vi "WLC Fitting_Final_v2_YCC.vi"(3 "initial parameters (Lp,Lc) or (Lc,K)":dbl[](array[numeric])=[40.0, 1150.0], 4 "Fitting Cluster":T1={"cr (um)"=0.0, "yr (V)"=0.0, "trap height(nm)"=300.0, "bead radius(nm)"=515.0, "Length offset"=550.0, "Upper Force(pN)"=500.0, "cr shift (nm)"=0.0, "yr shift (mV)"=0.0, "LaserPower (mW)"=1200.0, "conversion factor (V/um)"=0.0, "Stiffness (pN/nm)"=0.0, "xDNA cut outside"=3000.0, "Lower Force(pN)"=5.0, "c for zbd"=0.0}, 5 "Enum":T2(ring), 6 "Load Stage-QPD data":path, 7 "T=Fit U or twoside\nF=Fit F":bool=TRUE, 8 "F+U data?":bool, 9 "Finish Fitting":bool, 10 "Ready to Fit":bool, 11 "DataRecord type":enum32{"OneDirectionOnly?", "TwoSide Data"}(tab)) -> (0 "best fit parameters":dbl[](array[numeric]), 1 "r^2":dbl)   [LabVIEW 2014]
uses:
  <vilib>/gmath/NI_Gmath.lvlib
  <vilib>/gmath/NumericalOptimization/Nonlinear Curve Fit LM formula string.vi
  <vilib>/Utility/file.llb/Write To Spreadsheet File (DBL).vi
  <vilib>/Utility/file.llb/Read From Spreadsheet File (DBL).vi
  SubVI/WLC-Fitting Cluster.ctl
panel:
  in  "Given Lp (nm)":dbl=5.0
  in  "Lower Force (pN)":dbl=6.0
  in  "Upper Force (pN)":dbl=45.0
  in  "Set lower foce offset?":bool
  out "U-Force or twoside 2":dbl[](array[numeric])
  out "U-xDNA or twoside 2":dbl[](array[numeric])
  in  "initial guess K (pN)":dbl=1200.0
  out "OneDirectionOnly?":bool=TRUE
  in  "Fit \"+\"(RHS) ?":bool=TRUE
  in  "Fit One Side?":bool
  in  "Reverse sign?":bool=TRUE
  out "Cut-Force for eWLC (pN)":dbl[](array[numeric])
  out "best nonlinear fit extension (eWLC)":dbl[](array[numeric])
  in  "T=use stuckbead 7th order\nF=use slope 1st order calibrate":bool
  out "Force to be saved":dbl[](array[numeric])
  out "xDNA to be saved":dbl[](array[numeric])
  out "F-Force":dbl[](array[numeric])
  out "F-xDNA":dbl[](array[numeric])
  in  "F-yr shift (mV)":dbl
  in  "F-cr shift (nm)":dbl
  out "F-QPD signal (V)":dbl[](array[numeric])
  out "F-Stage Positions (um)":dbl[](array[numeric])
  in  "stuckbead path (dialog if empty)":path=path "D:/Calibration-Stuckbead-Scan/20181220/2/202224-x-Stuckbead Scan-6000.00-step 5.00 nm-QPD height 3.340-h0.txt"
  out "Save to Path":path
  out "best nonlinear fit force (M-S)":dbl[](array[numeric])
  in  "SaveName":enum16{"ForecExtension Only", "WLC Fitting"}(ring)
  in  "Save Calibrated Data?":bool
  out "U-Force or twoside":dbl[](array[numeric])
  out "U-xDNA or twoside":dbl[](array[numeric])
  out "Fitting Cluster for indicator":T1={"cr (um)"=0.0, "yr (V)"=0.0, "trap height(nm)"=0.0, "bead radius(nm)"=520.0, "Length offset"=0.0, "Upper Force(pN)"=0.0, "cr shift (nm)"=0.0, "yr shift (mV)"=0.0, "LaserPower (mW)"=0.0, "conversion factor (V/um)"=0.0, "Stiffness (pN/nm)"=0.0154, "xDNA cut outside"=0.0, "Lower Force(pN)"=5.0, "c for zbd"=0.0}
  in  "Tab Control":T3(tab)
  out "Stage-QPD Graph":T4(graph)
  out "U-Extension-Force Graph":cluster{"xDNA":dbl[], "Force":dbl[]}(graph)
  out "F-Extension-Force Graph":cluster{"xDNA":dbl[], "Force":dbl[]}(graph)
  out "All-Extension-Force Graph":T5(graph)
  out "Extension-Force and WLC Graph":cluster{"xDNA":dbl[], "Force":dbl[]}[](graph)
  out "All Extension-Force and WLC Graph":T6(graph)
  out "Cut Stage Position (um)":dbl[](array[numeric])
  out "Cut QPD (V)":dbl[](array[numeric])
  in  "Delete Outside Signal?":bool
  out "U-QPD signal or All QPD  (V)":dbl[](array[numeric])
  out "U-Stage Positions or All stage positions (um)":dbl[](array[numeric])
  in  "QPD":dbl[](array[numeric])
  in  "Stage":dbl[](array[numeric])
  in  "T=Read data mode?\nF=Real time fit":bool=TRUE
  # "5180bp=1750.8 nm\n3281bp=1109.0 nm"
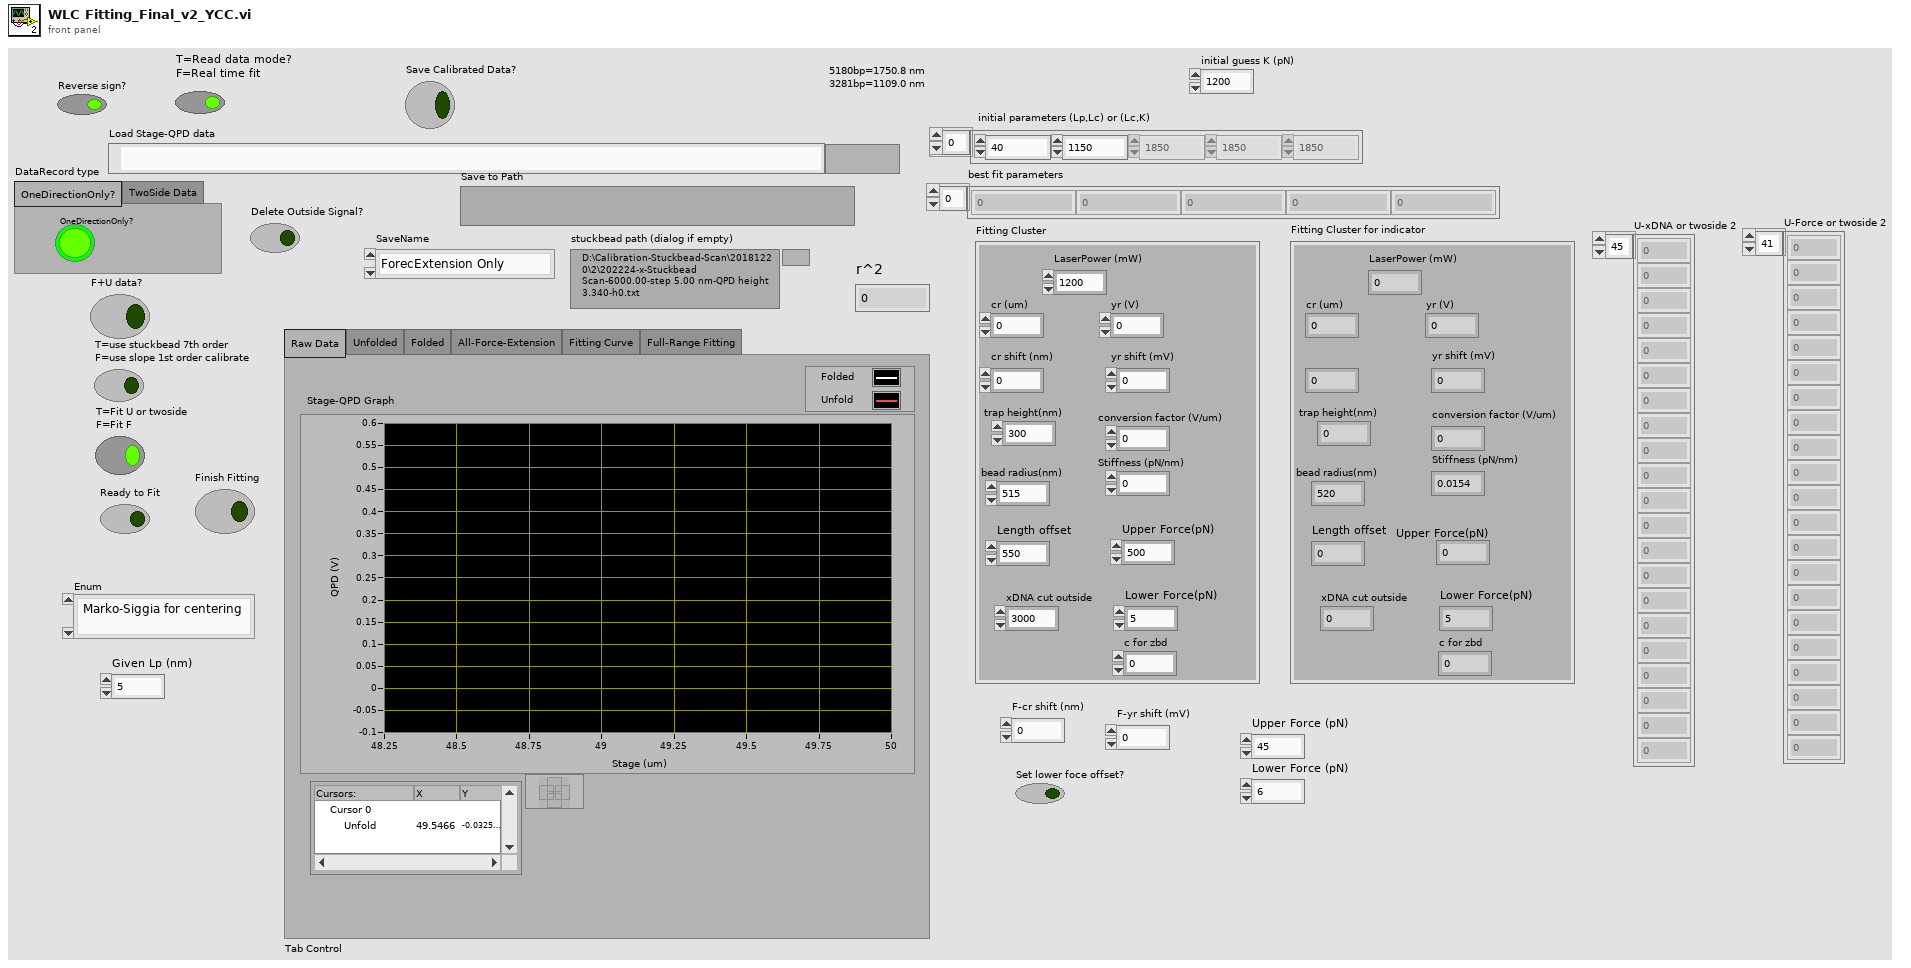
[diagram p1: front panel]
types:
  T1 = typedef "WLC-Fitting Cluster.ctl" = cluster{"cr (um)":dbl, "yr (V)":dbl, "trap height(nm)":dbl, "bead radius(nm)":dbl, "Length offset":dbl, "Upper Force(pN)":dbl, "cr shift (nm)":dbl, "yr shift (mV)":dbl, "LaserPower (mW)":dbl, "conversion factor (V/um)":dbl, "Stiffness (pN/nm)":dbl, "xDNA cut outside":dbl, "Lower Force(pN)":dbl, "c for zbd":dbl}
  T2 = enum16{" Marko-Siggia for centering", "Marko-Siggia", "direct fit (Lp,Lc,K)", "fit K (Lp,Lc,K)", "eWLC (Lp=45,Lc,K)"}
  T3 = enum32{"Raw Data", "Unfolded", "Folded", "All-Force-Extension", "Fitting Curve", "Full-Range Fitting"}
  T4 = cluster{"Sorted Stage Position (um)":dbl[], "Sorted QPD (V)":dbl[]}[]
  T5 = cluster{"Folded-xDNA":dbl[], "Folded-Force":dbl[]}[]
  T6 = cluster{"cut-full xDNA":dbl[], "cut-full Force":dbl[]}[]
  T7 = cluster{"model":string, "Parameters":string[], "x":string}
  T8 = cluster{"F-Stage Positions (um) ":dbl[], "F-QPD signal (V) ":dbl[]}
  T9 = cluster{"U-Stage Positions or All stage positions (um)":dbl[], "U-QPD signal or All QPD  (V)":dbl[]}
  T10 = cluster{"U-Stage Positions or All stage positions (um)":dbl[], "U-QPD signal or All QPD  (V)":dbl[]}[]
  T11 = cluster{"Folded-xDNA":dbl[], "Folded-xDNA":dbl[]}
  T12 = cluster{"cut-full xDNA":dbl[], "best nonlinear fit":dbl[]}
  T13 = cluster{"best nonlinear fit":dbl[], "cut-full Force":dbl[]}
  T14 = cluster{"cut-full xDNA":dbl[], "cut-full Force":dbl[]}
  T15 = cluster{"Fit Extension (nm)":dbl[], "Fit Force (pN)":dbl[]}
  T16 = cluster{"xDNA to be saved":dbl[], "Force to be saved":dbl[]}
  T17 = cluster{"xDNA to be saved":dbl[], "Force to be saved":dbl[]}[]
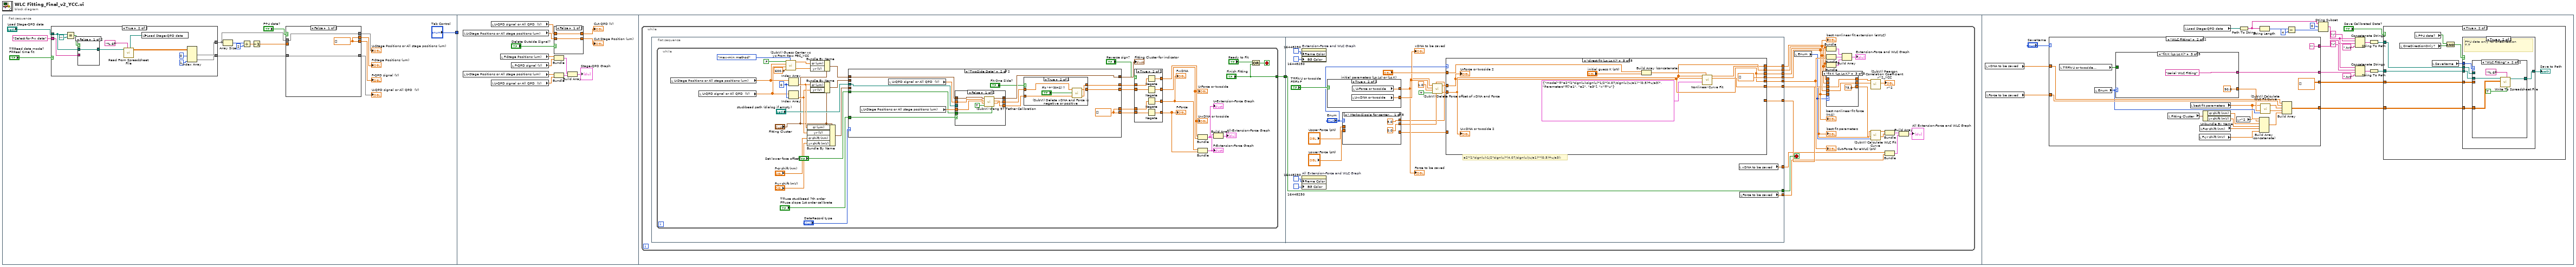
[diagram p0: block diagram]
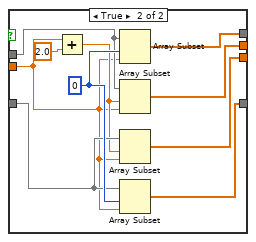
[diagram p2: hidden frame]
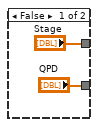
[diagram p3: hidden frame]
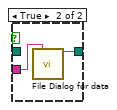
[diagram p4: hidden frame]
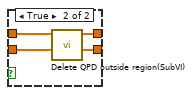
[diagram p5: hidden frame]
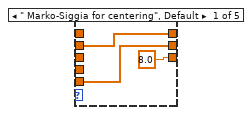
[diagram p6: hidden frame]
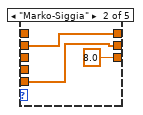
[diagram p7: hidden frame]
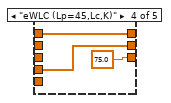
[diagram p8: hidden frame]
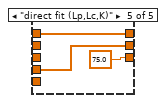
[diagram p9: hidden frame]
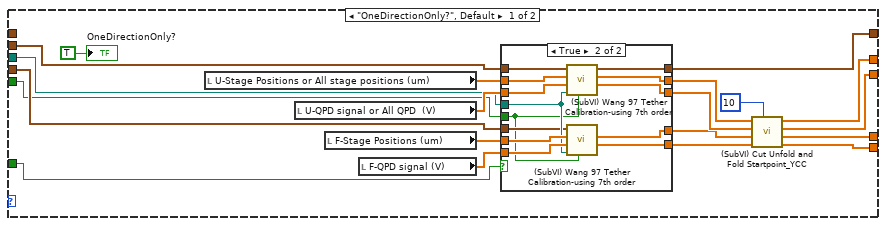
[diagram p11: hidden frame]
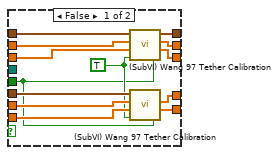
[diagram p12: hidden frame]
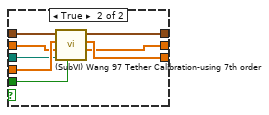
[diagram p14: hidden frame]
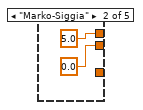
[diagram p15: hidden frame]
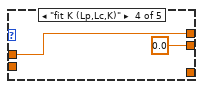
[diagram p17: hidden frame]
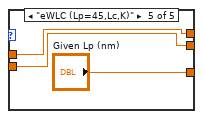
[diagram p18: hidden frame]
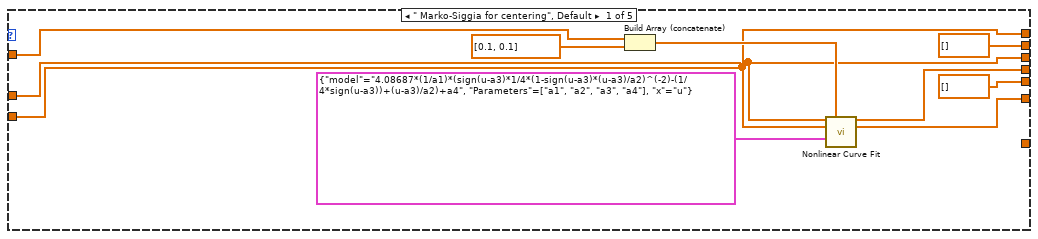
[diagram p19: hidden frame]
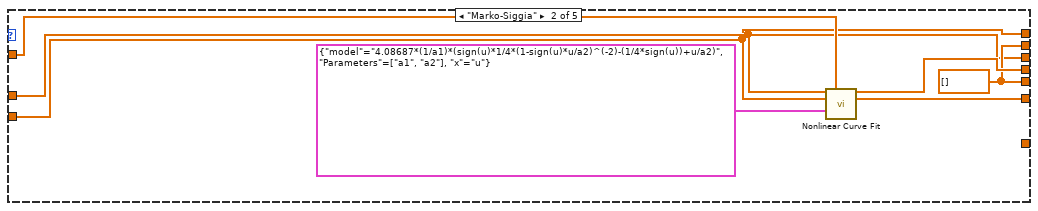
[diagram p20: hidden frame]
diagram:
  n1 = flat-sequence {
    tunnel: ["Tab Control"] -> w1
    tunnel: w1 -> [_]
    frame #0 {
      n2 = case shown="True" "T=Read data mode?\nF=Real time fit" {
        tunnel: ["QPD" w39] -> w11
        tunnel: ["Stage" w40] -> w6
        tunnel: "Select for F-x data" ("default name") -> [_ w36]
        tunnel: "Load Stage-QPD data" -> [_ w33]
        frame False {
        }
        frame True {
          n3 = Equal?(x=w33, y=path "") -> (x = y?=w34:bool)
          n4 = case shown="False" w34 {
            tunnel: [w44 w45] -> w37
            tunnel: w36 -> [_ w46]
            tunnel: w33 -> [w44 _]
            frame False {
            }
            frame True {
              n5 = call "File Dialog for data"("prompt"=w46) -> ("selected path"=w45:path)  [unwired: 11 in, 3 out]
            }
          }
          n6 = call-poly <vilib>:"Read From Spreadsheet File.vi"("format (%.3f)"="%.6f", "file path (dialog if empty)"=w37) -> ("all rows"=w43:dbl[][], "new file path (Not A Path if cancelled)"=w32:path)  [unwired: 5 in, 3 out]
          n7 = local write "Load Stage-QPD data"(w32) -> ()
          n8 = Index Array(array=w43, index (col) #1=0 ("disabled index (col)"), index (col) #2=1 ("index (col)")) -> (element #1=w40:dbl[], element #2=w39:dbl[])  [unwired: 2 in]
        }
      }
      n9 = Array Size(array=w6) -> (size(s)=w7:i32)
      n10 = Divide(x=w7, y=2) -> (x/y=w5:dbl)
      n11 = Decrement(x=w5) -> (x-1=w4:dbl)
      n12 = case shown="False" "F+U data?" {
        tunnel: w6 -> [w19 w25]
        tunnel: w11 -> [w18 w26]
        tunnel: [w19 w29] -> w10
        tunnel: [w18 w27] -> w9
        tunnel: w4 -> [_ w20]
        tunnel: [w17 w24] -> w3
        tunnel: [w17 w23] -> w2
        frame False {
          w17 = dbl[] []
        }
        frame True {
          w28 = 0 ("index")
          n13 = Add(x=w20, y=2.0) -> (x+y=w21:dbl)
          n14 = Array Subset(array=w25, index=w28, length=w20) -> (w29:dbl[])
          n15 = Array Subset(array=w25, index=w21, length=w20) -> (w24:dbl[])
          n16 = Array Subset(array=w26, index=w21, length=w20) -> (w23:dbl[])
          n17 = Array Subset(array=w26, index=w28, length=w20) -> (w27:dbl[])
        }
      }
      "U-Stage Positions or All stage positions (um)" <- w10
      "U-QPD signal or All QPD  (V)" <- w9
      "F-Stage Positions (um)" <- w3
      "F-QPD signal (V)" <- w2
    }
    frame #1 {
      n18 = local read "U-Stage Positions or All stage positions (um)"() -> (w57:dbl[])
      n19 = local read "U-Stage Positions or All stage positions (um)"() -> (w55:dbl[])
      n20 = local read "U-QPD signal or All QPD  (V)"() -> (w56:dbl[])
      n21 = local read "U-QPD signal or All QPD  (V)"() -> (w54:dbl[])
      n22 = local read "F-Stage Positions (um)"() -> (w48:dbl[])
      n23 = local read "F-QPD signal (V)"() -> (w47:dbl[])
      n24 = case shown="False" "Delete Outside Signal?" {
        tunnel: w56 -> [w60 w64]
        tunnel: w57 -> [w59 w63]
        tunnel: [w60 w62] -> w49
        tunnel: [w59 w61] -> w50
        frame False {
        }
        frame True {
          n25 = call "Delete QPD outside region(SubVI).vi"("Position Array In"=w63, "QPD signal In"=w64) -> ("Position Array Out"=w61:dbl[], "QPD signal Out"=w62:dbl[])  [unwired: 8 in]
        }
      }
      "Cut QPD (V)" <- w49
      "Cut Stage Position (um)" <- w50
      n26 = Bundle("F-Stage Positions (um)"=w48, "F-QPD signal (V)"=w47) -> (w53:T8)  [unwired: 1 in]
      n27 = Bundle("U-Stage Positions or All stage positions (um)"=w55, "U-QPD signal or All QPD  (V)"=w54) -> (w52:T9)  [unwired: 1 in]
      n28 = Build Array(w53, w52) -> (→"Stage-QPD Graph":T10)
    }
    frame #2 {
      n29 = while {
        stop <- w79 stop-if-true
        n30 = flat-sequence {
          tunnel: [w105] -> w80
          tunnel: [w262] -> w85
          tunnel: [w261] -> w76
          tunnel: [w259] -> w82
          tunnel: [w258] -> w86
          tunnel: [w257] -> w81
          tunnel: [w256] -> w88
          tunnel: [w255] -> w79
          tunnel: w80 -> [w255]
          tunnel: [w242] -> w77
          tunnel: [w241] -> w68
          tunnel: [w240] -> w67
          frame #0 {
            n31 = while {
              tunnel: ["Finish Fitting"] -> w105
              stop <- w109 stop-if-true
              w141 = 0 ("index")
              n32 = local read "U-Stage Positions or All stage positions (um)"() -> (w130:dbl[])
              n33 = local read "U-QPD signal or All QPD  (V)"() -> (w129:dbl[])
              n34 = call "(SubVI) Guess Center xc yc From Raw FEC_YCC.vi"("Read data?"=FALSE, "Enum"=enum16{"parity method", "max-min method"}."max-min method", "Stage array(um)"=w130, "QPD array (V)"=w129, "avg range for QPD center (nm)"=600.0) -> ("Guess-stage-center (um)"=w128:dbl, "Guess-QPD-center (V)"=w127:dbl)  [unwired: 2 in]
              n35 = Index Array(array=w130, index=w141) -> (element=w138:dbl)
              n36 = Index Array(array=w129, index=w141) -> (element=w137:dbl)
              n37 = Bundle By Name(cluster="Fitting Cluster", "cr (um)"=w138, "yr (V)"=w137, "cr shift (nm)"="F-cr shift (nm)", "yr shift (mV)"="F-yr shift (mV)") -> (w134:T1)
              n38 = Bundle By Name(cluster="Fitting Cluster", "cr (um)"=w128, "yr (V)"=w127) -> (w126:T1)
              n39 = Bundle By Name(cluster="Fitting Cluster", "cr (um)"=w138, "yr (V)"=w137) -> (w140:T1)
              n40 = case shown="\"TwoSide Data\"" "DataRecord type" {
                tunnel: w140 -> [w171 _]
                tunnel: [w172 w209] -> w139
                tunnel: w134 -> [w167 _]
                tunnel: w126 -> [_ w212]
                tunnel: [w161 w202] -> w123
                tunnel: [w160 w201] -> w117
                tunnel: [w159 w208] -> w122
                tunnel: [w158 w208] -> w121
                tunnel: "T=use stuckbead 7th order\nF=use slope 1st order calibrate" -> [w157 w207]
                tunnel: "stuckbead path (dialog if empty)" -> [w156 w206]
                tunnel: "Set lower foce offset?" -> [w154 w200]
                frame "OneDirectionOnly?", Default {
                  n41 = local read "U-Stage Positions or All stage positions (um)"() -> (w170:dbl[])
                  n42 = local read "U-QPD signal or All QPD  (V)"() -> (w173:dbl[])
                  n43 = local read "F-Stage Positions (um)"() -> (w169:dbl[])
                  n44 = local read "F-QPD signal (V)"() -> (w168:dbl[])
                  n45 = case shown="True" w157 {
                    tunnel: w173 -> [w185 w199]
                    tunnel: [w184 w198] -> w172
                    tunnel: w171 -> [w176 w197]
                    tunnel: w170 -> [w186 w196]
                    tunnel: w169 -> [w182 w195]
                    tunnel: w168 -> [w181 w194]
                    tunnel: w156 -> [_ w193]
                    tunnel: w167 -> [w183 w192]
                    tunnel: [w180 w191] -> w165
                    tunnel: [w179 w190] -> w164
                    tunnel: [w178 w189] -> w163
                    tunnel: [w177 w188] -> w162
                    tunnel: w154 -> [w174 w187]
                    frame False {
                      w175 = TRUE ("X=T\nY=F")
                      n46 = call "(SubVI) Wang 97 Tether Calibration.vi"("Set lower foce offset?"=w174, "X=T\nY=F"=w175, "QPD signal"=w185, "Stage Position"=w186, "Fitting Cluster"=w176) -> ("Force"=w179:dbl[], "xDNA"=w180:dbl[], "output cluster"=w184:T1)
                      n47 = call "(SubVI) Wang 97 Tether Calibration.vi"("Set lower foce offset?"=w174, "X=T\nY=F"=w175, "QPD signal"=w181, "Stage Position"=w182, "Fitting Cluster"=w183) -> ("Force"=w177:dbl[], "xDNA"=w178:dbl[])  [unwired: 1 out]
                    }
                    frame True {
                      n48 = call "(SubVI) Wang 97 Tether Calibration-using 7th order.vi"("Set lower foce offset?"=w187, "stuckbead path (dialog if empty)"=w193, "QPD signal"=w199, "Stage Position"=w196, "Fitting Cluster"=w197) -> ("Force"=w190:dbl[], "xDNA"=w191:dbl[], "output cluster"=w198:T1)  [unwired: 2 in, 2 out]
                      n49 = call "(SubVI) Wang 97 Tether Calibration-using 7th order.vi"("Set lower foce offset?"=w187, "stuckbead path (dialog if empty)"=w193, "QPD signal"=w194, "Stage Position"=w195, "Fitting Cluster"=w192) -> ("Force"=w188:dbl[], "xDNA"=w189:dbl[])  [unwired: 2 in, 3 out]
                    }
                  }
                  n50 = call "(SubVI) Cut Unfold and Fold Startpoint_YCC.vi"("number to cut"=10, "Folded-Force in"=w162, "Folded-xDNA in"=w163, "Unfolded-Force"=w164, "Unfolded-xDNA"=w165) -> ("Folded-Force"=w158:dbl[], "Folded-xDNA"=w159:dbl[], "Unfolded-Force"=w160:dbl[], "Unfolded-xDNA"=w161:dbl[])  [unwired: 3 in]
                  "OneDirectionOnly?" <- TRUE
                }
                frame "TwoSide Data" {
                  w208 = dbl[] [] ("Folded-xDNA")
                  n51 = local read "U-Stage Positions or All stage positions (um)"() -> (w211:dbl[])
                  n52 = local read "U-QPD signal or All QPD  (V)"() -> (w210:dbl[])
                  n53 = case shown="False" w207 {
                    tunnel: w212 -> [w227 w235]
                    tunnel: w211 -> [w226 w234]
                    tunnel: w210 -> [w225 w233]
                    tunnel: [w224 w231] -> w209
                    tunnel: [w223 w230] -> w203
                    tunnel: [w222 w229] -> w204
                    tunnel: w206 -> [_ w232]
                    tunnel: w200 -> [w220 w228]
                    frame False {
                      n54 = call "(SubVI) Wang 97 Tether Calibration.vi"("Set lower foce offset?"=w220, "X=T\nY=F"=TRUE ("X=T\nY=F"), "QPD signal"=w225, "Stage Position"=w226, "Fitting Cluster"=w227) -> ("Force"=w222:dbl[], "xDNA"=w223:dbl[], "output cluster"=w224:T1)
                    }
                    frame True {
                      n55 = call "(SubVI) Wang 97 Tether Calibration-using 7th order.vi"("Set lower foce offset?"=w228, "stuckbead path (dialog if empty)"=w232, "QPD signal"=w233, "Stage Position"=w234, "Fitting Cluster"=w235) -> ("Force"=w229:dbl[], "xDNA"=w230:dbl[], "output cluster"=w231:T1)  [unwired: 2 in, 2 out]
                    }
                  }
                  n56 = case shown="True" "Fit One Side?" {
                    tunnel: w204 -> [w214 w218]
                    tunnel: w203 -> [w213 w217]
                    tunnel: [w213 w216] -> w202
                    tunnel: [w214 w215] -> w201
                    frame False {
                    }
                    frame True {
                      n57 = call "(SubVI) Delete xDNA and Force is negative or positive.vi"("xDNA"=w217, "T=positive (RHS)\nF=negative (LHS)"="Fit \"+\"(RHS) ?", "Force"=w218) -> ("xDNA-cut"=w216:dbl[], "Force-cut"=w215:dbl[])  [unwired: 1 in]
                    }
                  }
                }
              }
              "Fitting Cluster for indicator" <- w139
              n58 = case shown="True" "Reverse sign?" {
                tunnel: w123 -> [w145 w147]
                tunnel: w122 -> [w143 w153]
                tunnel: w121 -> [w142 w152]
                tunnel: [w142 w151] -> w120
                tunnel: [w143 w150] -> w119
                tunnel: [w145 w146] -> w118
                tunnel: w117 -> [w144 w149]
                tunnel: [w144 w148] -> w116
                frame False {
                }
                frame True {
                  n59 = Negate(x=w147) -> (-x=w146:dbl[])
                  n60 = Negate(x=w149) -> (-x=w148:dbl[])
                  n61 = Negate(x=w153) -> (-x=w150:dbl[])
                  n62 = Negate(x=w152) -> (-x=w151:dbl[])
                }
              }
              "U-xDNA or twoside" <- w118
              "U-Force or twoside" <- w116
              "F-xDNA" <- w119
              "F-Force" <- w120
              n63 = Bundle("xDNA-cut"=w118, "Force-cut"=w116) -> (w131:cluster{"xDNA-cut":dbl[], "Force-cut":dbl[]})  [unwired: 1 in]
              "U-Extension-Force Graph" <- w131
              n64 = Bundle("Folded-xDNA"=w119, "Folded-xDNA"=w120) -> (w132:T11)  [unwired: 1 in]
              "F-Extension-Force Graph" <- w132
              n65 = Build Array(w132, w131) -> (→"All-Extension-Force Graph":cluster{"xDNA-cut":dbl[], "Force-cut":dbl[]}[])
              n66 = Or(x="Ready to Fit", y="Finish Fitting") -> (x .or. y?=w109:bool)
            }
          }
          frame #1 {
            # "a2*(1*sign(u)-1/2*sign(u)*(4.07/sign(u)/u/a1)**(0.5)+u/a3);"
            n67 = property on="Extension-Force and WLC Graph" class="XYGraph (strict)"("Frame Color"=u32 16448250, "BG Color"=u32 16448250) -> ()  [unwired: 2 in, 2 out]
            n68 = property on="All Extension-Force and WLC Graph" class="XYGraph (strict)"("Frame Color"=u32 16448250, "BG Color"=u32 16448250) -> ()  [unwired: 2 in, 2 out]
            n69 = case shown="True" "T=Fit U or twoside\nF=Fit F" {
              tunnel: [w329 w331] -> w250
              tunnel: [w328 w330] -> w249
              frame False {
                n70 = local read "F-xDNA"() -> (w329:dbl[])
                n71 = local read "F-Force"() -> (w328:dbl[])
              }
              frame True {
                n72 = local read "U-xDNA or twoside"() -> (w331:dbl[])
                n73 = local read "U-Force or twoside"() -> (w330:dbl[])
              }
            }
            "xDNA to be saved" <- w250
            "Force to be saved" <- w249
            n74 = case shown="\" Marko-Siggia for centering\", Default" "Enum" {
              tunnel: [0.0 0.0 w268 0.0 ("Lower Force (pN)") w273] -> w247
              tunnel: [5.0 5.0 w269 w270 w274] -> w246
              tunnel: "Upper Force (pN)" -> [_ _ w269 w270 w274]
              tunnel: "Lower Force (pN)" -> [_ _ w268 _ w273]
              tunnel: [_ _ _ _ "Given Lp (nm)"] -> w243
              frame " Marko-Siggia for centering", Default {
              }
              frame "Marko-Siggia" {
              }
              frame "direct fit (Lp,Lc,K)" {
              }
              frame "fit K (Lp,Lc,K)" {
              }
              frame "eWLC (Lp=45,Lc,K)" {
              }
            }
            n75 = call "(SubVI) Delete Force offset of xDNA and Force.vi"("Force"=w249, "Upper Force (pN)"=w246, "xDNA"=w250, "force constant"=1.0, "Lower Force (pN)"=w247, "Set lower foce offset?"=TRUE) -> ("cut-full Force"=w251:dbl[], "cut-full xDNA"=w252:dbl[])  [unwired: 1 in]
            n76 = case shown="\"direct fit (Lp,Lc,K)\"" "Enum" {
              tunnel: "initial parameters (Lp,Lc) or (Lc,K)" -> [w281 w288 w305 _ w326]
              tunnel: w251 -> [w275 w286 w301 w316 w320]
              tunnel: w252 -> [w276 w285 w302 w308 w322]
              tunnel: [w279 w290 dbl[] [] ("best nonlinear fit") dbl[] [] ("best nonlinear fit") dbl[] [] ("best nonlinear fit")] -> w262
              tunnel: [w280 w289 w299 w306 w324] -> w261
              tunnel: [w276 w285 w302 w308 w322] -> w259
              tunnel: [w275 w286 w301 w316 w320] -> w258
              tunnel: [dbl[] [] ("best nonlinear fit extension for eWLC") w287 w304 w314 w323] -> w257
              tunnel: [dbl[] [] ("Cut-Force (pN)") w287 w301 w312 w320] -> w256
              tunnel: w243 -> [_ _ w292 _ _]
              tunnel: [_ _ _ w307 _] -> w242
              frame " Marko-Siggia for centering", Default {
                n77 = Build Array (concatenate)(w281, dbl[] [0.1, 0.1] ("element")) -> (w282:dbl[])
                n78 = call-poly <vilib>:"Nonlinear Curve Fit.vi"("Y"=w275, "initial parameters"=w282, "X"=w276, "model description"=T7 {"model"="4.08687*(1/a1)*(sign(u-a3)*1/4*(1-sign(u-a3)*(u-a3)/a2)^(-2)-(1/4*sign(u-a3))+(u-a3)/a2)+a4", "Parameters"=["a1", "a2", "a3", "a4"], "x"="u"}) -> ("best nonlinear fit"=w279:dbl[], "best fit parameters"=w280:dbl[])  [unwired: 3 in, 7 out]
              }
              frame "Marko-Siggia" {
                w287 = dbl[] [] ("best nonlinear fit extension for eWLC")
                n79 = call-poly <vilib>:"Nonlinear Curve Fit.vi"("Y"=w286, "initial parameters"=w288, "X"=w285, "model description"=T7 {"model"="4.08687*(1/a1)*(sign(u)*1/4*(1-sign(u)*u/a2)^(-2)-(1/4*sign(u))+u/a2)", "Parameters"=["a1", "a2"], "x"="u"}) -> ("best nonlinear fit"=w290:dbl[], "best fit parameters"=w289:dbl[])  [unwired: 3 in, 7 out]
              }
              frame "eWLC (Lp=45,Lc,K)" {
                n80 = Number To Decimal String(number=w292) -> (decimal integer string=w298:string)  [unwired: 1 in]
                n81 = Concatenate Strings("a1*(1*sign(u)-sign(u)*1/2*(4.07/sign(u)/u/" ("model"), w298, ")^(0.5)+u/a2)" ("model")) -> (w294:string)
                n82 = Bundle(cluster=T7 {"model"="a1*(1*sign(u)-sign(u)*1/2*(4.07/sign(u)/u/45)^(0.5)+u/a2)", "Parameters"=["a1", "a2"], "x"="u"} ("model description"), "model"=w294) -> (w293:T7)  [unwired: 2 in]
                n83 = call-poly <vilib>:"Nonlinear Curve Fit.vi"("Y"=w302, "initial parameters"=w305, "X"=w301, "model description"=w293) -> ("best nonlinear fit"=w304:dbl[], "best fit parameters"=w300:dbl[])  [unwired: 3 in, 7 out]
                n84 = Build Array (concatenate)(w292, w300) -> (w299:dbl[])
              }
              frame "fit K (Lp,Lc,K)" {
                n85 = call "Serial fit Lc and K.vi"("Extension (nm)"=w308, "Force (pN)"=w316, "initial parameters for WLC (Lp,Lc)"=dbl[] [45.0, 1200.0], 5:dbl[] [1200.0, 1200.0] ("initial parameters for eWLC (Lc,K)")) -> ("Cut-Extenison (nm)"=w307:dbl[], "Cut-Force (pN)"=w312:dbl[], "best fit parameters for eWLC (Lp,Lc,K)"=w306:dbl[], "best fit parameters for WLC"=w315:dbl[], "best nonlinear fit extension for eWLC"=w314:dbl[])
                n86 = Delete From Array(array=w306, length=1, index=0) -> (array with subset deleted=w309:dbl[])  [unwired: 1 out]
                n87 = Build Array (concatenate)(w315, w309) -> ()  [unwired: 1 out]
              }
              frame "direct fit (Lp,Lc,K)" {
                n88 = Build Array (concatenate)(w326, "initial guess K (pN)") -> (w325:dbl[])
                n89 = call-poly <vilib>:"Nonlinear Curve Fit.vi"("Y"=w322, "initial parameters"=w325, "X"=w320, "model description"=T7 {"model"="a2*(1*sign(u)-sign(u)*1/2*(4.07/sign(u)/u/a1)^(0.5)+u/a3)", "Parameters"=["a1", "a2", "a3"], "x"="u"}) -> ("best nonlinear fit"=w323:dbl[], "best fit parameters"=w324:dbl[])  [unwired: 3 in, 7 out]
                "U-xDNA or twoside 2" <- w322
                "U-Force or twoside 2" <- w320
              }
            }
            n90 = local read "xDNA to be saved"() -> (w241:dbl[])
            n91 = local read "Force to be saved"() -> (w240:dbl[])
          }
        }
        n92 = local read "Enum"() -> (w75:T2)
        n93 = Bundle("cut-full xDNA"=w82, "best nonlinear fit"=w85) -> (w89:T12)  [unwired: 1 in]
        n94 = Bundle("best nonlinear fit"=w81, "cut-full Force"=w88) -> (w78:T13)  [unwired: 1 in]
        n95 = Bundle("cut-full xDNA"=w82, "cut-full Force"=w86) -> (w72:T14)  [unwired: 1 in]
        n96 = case shown="\"fit K (Lp,Lc,K)\"" w75 {
          tunnel: w86 -> [w92 w95 _ _ _]
          tunnel: w85 -> [w91 w94 _ _ _]
          tunnel: [w92 w95 w97 w101 w103] -> w84
          tunnel: [w91 w94 w98 w100 w104] -> w83
          tunnel: w82 -> [_ _ _ w101 w103]
          tunnel: w81 -> [_ _ w98 w100 w104]
          tunnel: w77 -> [_ _ w97 _ _]
          tunnel: [8.0 ("Force Upper Limit") 8.0 ("Force Upper Limit") 75.0 ("Force Upper Limit") 75.0 ("Force Upper Limit") 75.0 ("Force Upper Limit")] -> w65
          frame " Marko-Siggia for centering", Default {
          }
          frame "Marko-Siggia" {
          }
          frame "fit K (Lp,Lc,K)" {
          }
          frame "eWLC (Lp=45,Lc,K)" {
          }
          frame "direct fit (Lp,Lc,K)" {
          }
        }
        n97 = Build Array(w89, w78, w72) -> (→"Extension-Force and WLC Graph":T6)
        n98 = call "(SubVI) Pearson Correlation Coefficient r^2_YCC.vi"("best fit Data"=w83, "Data"=w84) -> ("r^2"=→"r^2":dbl)  [unwired: 4 in, 1 out]
        n99 = call "(SubVI) Calculate WLC Fit Curve.vi"("Enum 2"=w75, "Force Upper Limit"=w65, "BestFit"=w76) -> ("Fit Force (pN)"=w73:dbl[], "Fit Extension (nm)"=w74:dbl[])  [unwired: 4 in]
        n100 = Bundle("Fit Extension (nm)"=w74, "Fit Force (pN)"=w73) -> (w71:T15)  [unwired: 1 in]
        n101 = Bundle("xDNA to be saved"=w68, "Force to be saved"=w67) -> (w66:T16)  [unwired: 1 in]
        n102 = Build Array(w71, w66) -> (→"All Extension-Force and WLC Graph":T17)
        "best nonlinear fit force (M-S)" <- w85
        "best fit parameters" <- w76
        "best nonlinear fit extension (eWLC)" <- w81
        "Cut-Force for eWLC (pN)" <- w88
      }
    }
    frame #3 {
      n103 = local read "xDNA to be saved"() -> (w333:dbl[])
      n104 = local read "Force to be saved"() -> (w332:dbl[])
      n105 = case shown="\"WLC Fitting\"" "SaveName" {
        tunnel: [w363 w383] -> w345
        tunnel: [w362 w399] -> w342
        tunnel: [w361 "" ("string")] -> w337
        tunnel: [w360 dbl[][] []] -> w334
        tunnel: w333 -> [w357 w396]
        tunnel: w332 -> [w356 w395]
        frame "ForecExtension Only", Default {
          n106 = local read "OneDirectionOnly?"() -> (w355:bool)
          n107 = local read "F+U data?"() -> (w359:bool)
          n108 = And(x=w359, y=w355) -> (x .and. y?=w358:bool)
          n109 = case shown="True" w358 {
            tunnel: [w370 "U-ForecExtension Only" ("string")] -> w363
            tunnel: [w367 w377] -> w362
            tunnel: ["" ("string") "F-ForecExtension Only" ("string")] -> w361
            tunnel: [dbl[][] [] w373] -> w360
            tunnel: w357 -> [w366 _]
            tunnel: w356 -> [w365 _]
            tunnel: w355 -> [w364 _]
            frame False {
              n110 = case shown="True" w364 {
                tunnel: ["twoside-ForecExtension Only" ("string") "U-ForecExtension Only" ("string")] -> w370
                frame False {
                }
                frame True {
                }
              }
              n111 = Build Array(w366, w365) -> (w367:dbl[][])
            }
            frame True {
              n112 = local read "U-xDNA or twoside"() -> (w379:dbl[])
              n113 = local read "U-Force or twoside"() -> (w378:dbl[])
              n114 = local read "F-xDNA"() -> (w376:dbl[])
              n115 = local read "F-Force"() -> (w375:dbl[])
              n116 = Build Array(w376, w375) -> (w373:dbl[][])
              n117 = Build Array(w379, w378) -> (w377:dbl[][])
            }
          }
        }
        frame "WLC Fitting" {
          n118 = local read "T=Fit U or twoside\nF=Fit F"() -> (w382:bool)
          n119 = local read "Enum"() -> (w392:T2)
          n120 = case shown="\"fit K (Lp,Lc,K)\"" w392 {
            tunnel: [90.0 ("Force Upper Limit") 90.0 ("Force Upper Limit") 90.0 ("Force Upper Limit") 150.0 ("Force Upper Limit") 90.0 ("Force Upper Limit")] -> w394
            tunnel: ["MS-WLC Fitting" ("string") "MS-WLC Fitting" ("string") "serial WLC Fitting" ("string") "eWLC Fitting Lp45" ("string") w409] -> w383
            tunnel: w382 -> [_ _ _ _ w408]
            frame " Marko-Siggia for centering", Default {
            }
            frame "Marko-Siggia" {
            }
            frame "fit K (Lp,Lc,K)" {
            }
            frame "eWLC (Lp=45,Lc,K)" {
            }
            frame "direct fit (Lp,Lc,K)" {
              n121 = case shown="False" w408 {
                tunnel: ["Folded-eWLC Fitting" ("string") "Unfolded-eWLC Fitting" ("string")] -> w409
                frame False {
                }
                frame True {
                }
              }
            }
          }
          n122 = local read "Fitting Cluster"() -> (w388:T1)
          n123 = local read "best fit parameters"() -> (w391:dbl[])
          n124 = local read "F-yr shift (mV)"() -> (w384:dbl)
          n125 = local read "F-cr shift (nm)"() -> (w385:dbl)
          n126 = Unbundle By Name(w388) -> ("cr shift (nm)"=w387:dbl, "yr shift (mV)"=w386:dbl)
          n127 = local read "r^2"() -> (w390:dbl)
          n128 = Build Array (concatenate)(w391, w390, w387, w386, w385, w384) -> (w389:dbl[])
          n129 = call "(SubVI) Calculate WLC Fit Curve.vi"("Enum 2"=w392, "Force Upper Limit"=w394, "BestFit"=w391) -> ("Fit Force (pN)"=w393:dbl[], "Fit Extension (nm)"=w381:dbl[])  [unwired: 4 in]
          n130 = Build Array(w396, w395, w381, w393, w389) -> (w399:dbl[][])
        }
      }
      n131 = local read "Load Stage-QPD data"() -> (w354:path)
      n132 = Path To String(path=w354) -> (string=w352:string)
      n133 = String Length(string=w352) -> (length=w351:i32)
      n134 = Subtract(x=w351, y=4) -> (x-y=w348:i32)
      n135 = String Subset(string=w352, offset (0)=0, length (rest)=w348) -> (substring=w339:string)
      n136 = Concatenate Strings(w339, "-" ("string"), w337, ".txt" ("string")) -> (w340:string)
      n137 = Concatenate Strings(w339, "-" ("string"), w345, ".txt" ("string")) -> (w341:string)
      n138 = String To Path(string=w340) -> (path=w335:path)
      n139 = String To Path(string=w341) -> (path=w343:path)
      n140 = case shown="True" "Save Calibrated Data?" {
        tunnel: w343 -> [_ w421]
        tunnel: w342 -> [_ w420]
        tunnel: w335 -> [_ w419]
        tunnel: w334 -> [_ w418]
        frame False {
        }
        frame True {
          n141 = local read "OneDirectionOnly?"() -> (w416:bool)
          n142 = local read "F+U data?"() -> (w415:bool)
          n143 = local read "SaveName"() -> (w413:enum16{"ForecExtension Only", "WLC Fitting"})
          n144 = And(x=w415, y=w416) -> (x .and. y?=w414:bool)
          n145 = case shown="True" w414 {
            tunnel: w421 -> [w423 w432]
            tunnel: w420 -> [w424 w431]
            tunnel: w419 -> [_ w430]
            tunnel: w418 -> [_ w429]
            tunnel: [w422 w428] -> w417
            tunnel: w413 -> [_ w427]
            frame False {
              # "twoside data or Unfolded data only"
              n146 = call-poly <vilib>:"Write To Spreadsheet File.vi"("transpose? (no:F)"=TRUE, "format (%.3f)"="%.6f", "2D data"=w424, "file path (dialog if empty)"=w423) -> ("new file path (Not A Path if cancelled)"=w422:path)  [unwired: 4 in]
            }
            frame True {
              # "F+U data only for onedirection\nT,T"
              n147 = case shown="\"WLC Fitting\"" w427 {
                tunnel: w432 -> [w440 w442]
                tunnel: w431 -> [w439 w443]
                tunnel: w430 -> [w436 _]
                tunnel: w429 -> [w435 _]
                tunnel: [w433 w441] -> w428
                frame "ForecExtension Only", Default {
                  w437 = "%.6f" ("format (%.3f)")
                  n148 = call-poly <vilib>:"Write To Spreadsheet File.vi"("transpose? (no:F)"=TRUE, "format (%.3f)"=w437, "2D data"=w435, "file path (dialog if empty)"=w436) -> ()  [unwired: 4 in, 1 out]
                  n149 = call-poly <vilib>:"Write To Spreadsheet File.vi"("transpose? (no:F)"=TRUE, "format (%.3f)"=w437, "2D data"=w439, "file path (dialog if empty)"=w440) -> ("new file path (Not A Path if cancelled)"=w433:path)  [unwired: 4 in]
                }
                frame "WLC Fitting" {
                  n150 = call-poly <vilib>:"Write To Spreadsheet File.vi"("transpose? (no:F)"=TRUE, "format (%.3f)"="%.6f", "2D data"=w443, "file path (dialog if empty)"=w442) -> ("new file path (Not A Path if cancelled)"=w441:path)  [unwired: 4 in]
                }
              }
            }
          }
          "Save to Path" <- w417
        }
      }
    }
  }
